vi "ADAM_Hi-Tec_convert.vi"(0 "Ch Name":string, 1 "Raw":dbl format="%.3f") -> (5 "Q release (l/min)":dbl format="%.2f", 6 "M_dot (kg/min)":dbl format="%.4f", 7 "Comments":string)   [LabVIEW 2015]
uses:
  Anemometry/Anemometry Sub Vis/Globals/Gas_management_global.vi
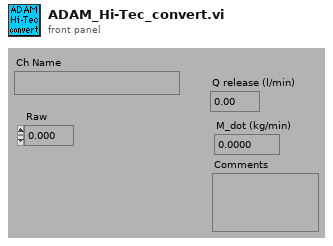
[diagram p1: front panel]
types:
  T1 = enum16{"Q(release) to Volts", "Volts to Q(release)"}
  T2 = typedef "Hi-Tec_calib.ctl" = cluster{"Ref temp (deg C)":dbl, "Ref Pres (mbars)":dbl, "Density at calib conditions":dbl, "Coefficients":dbl[]}
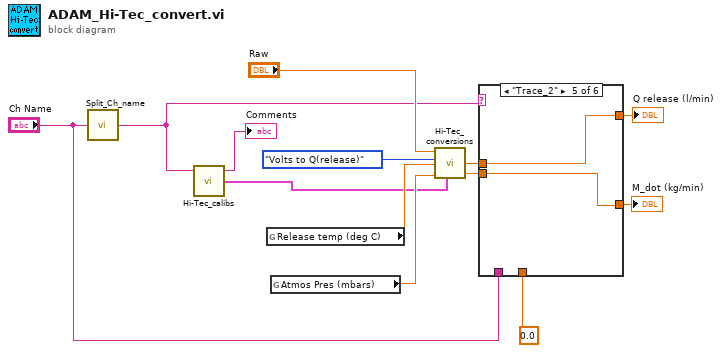
[diagram p0: block diagram]
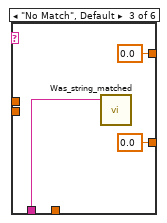
[diagram p4: hidden frame]
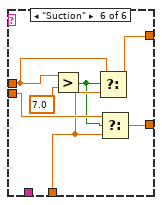
[diagram p6: hidden frame]
diagram:
  n1 = call "Split_Ch_name.vi"("Ch name"="Ch Name") -> ("Middle"=w3:string)  [unwired: 2 out]
  n2 = call "Hi-Tec_calibs.vi"("Gas Line Name"=w3) -> ("Hi-Tec calib"=w5:T2, "Comments"=→"Comments":string)  [unwired: 3 out]
  n3 = global read "Gas_management_global.vi" "Release temp (deg C)"() -> (w12:dbl)
  n4 = global read "Gas_management_global.vi" "Atmos Pres (mbars)"() -> (w11:dbl)
  n5 = call "Hi-Tec_conversions.vi"("Input"="Raw", "Conversion"=T1."Volts to Q(release)", "Release temp (deg C)"=w12, "Atmos Pres (mbars)"=w11, "Hi-Tec calib"=w5) -> ("Output"=w9:dbl, "Flowrate (kg/min)"=w7:dbl)  [unwired: 1 out]
  n6 = case shown="\"Trace_2\"" w3 {
    tunnel: w9 -> [w15 w17 _ w22 w24 w27]
    tunnel: [w15 w17 0.0 ("Output") w22 w24 w31] -> w8
    tunnel: w7 -> [w14 w16 _ w21 w23 w30]
    tunnel: [w14 w16 0.0 ("Flowrate (kg/min)") w21 w23 w29] -> w6
    tunnel: 0.0 -> [_ _ _ _ _ w28]
    tunnel: "Ch Name" -> [_ _ w20 _ _ _]
    frame "Carrier 1" {
    }
    frame "Carrier 2" {
    }
    frame "No Match", Default {
      n7 = call "Was_string_matched.vi"("Variable name"=w20) -> ()  [unwired: 2 in]
    }
    frame "Trace" {
    }
    frame "Trace_2" {
    }
    frame "Suction" {
      n8 = Greater?(x=w27, y=7.0) -> (0:w26:bool)
      n9 = Select(t=w27, s=w26, f=w28) -> (s? t:f=w31:dbl)
      n10 = Select(t=w30, s=w26, f=w28) -> (s? t:f=w29:dbl)
    }
  }
  "Q release (l/min)" <- w8
  "M_dot (kg/min)" <- w6
